vi "Open Session.vi"(6 "verify server (T)":bool=TRUE, 8 "error in":errorcluster, 9 "password":string, 10 "username":string, 11 "cookie file":path) -> (0 "error out":errorcluster, 3 "session":refnum<class "Session.lvclass">)   [LabVIEW 2024, in "lib_NI_Advanced HTTP Client.lvlib" / "Session.lvclass"]
doc: "Opens an HTTP client session. Use an HTTP client session to wire together multiple HTTP VIs while preserving authentication credentials, HTTP headers, and cookies."
uses:
  Session.lvclass
  Session.lvclass/Session.ctl
  lvwebclient_64.dll
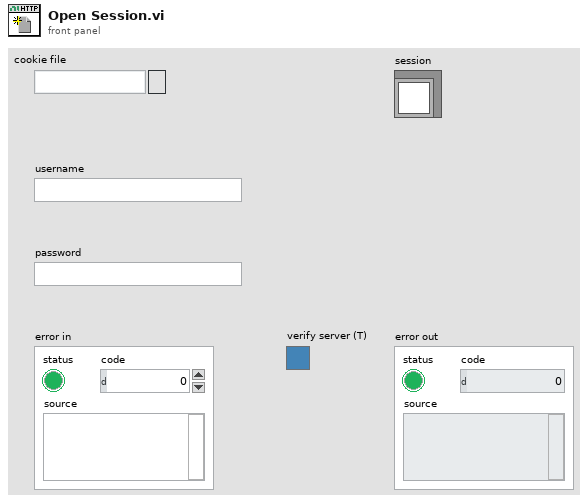
[diagram p1: front panel]
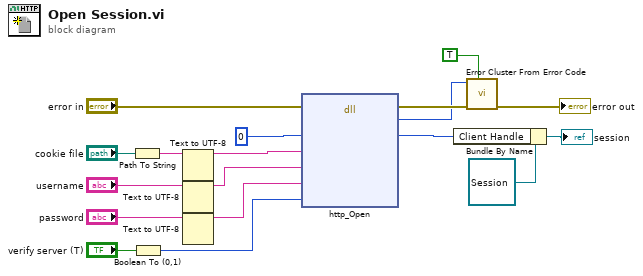
[diagram p0: block diagram]
diagram:
  n1 = Path To String(path="cookie file") -> (string=w6:string)
  n2 = Boolean To (0,1)(Boolean="verify server (T)") -> (0, 1=w12:i16)
  n3 = Text to UTF-8(11:w6) -> (3:w1:string)  [unwired: 2 in, 1 out]
  n4 = Text to UTF-8(11:"username") -> (3:w2:string)  [unwired: 2 in, 1 out]
  n5 = Text to UTF-8(11:"password") -> (3:w3:string)  [unwired: 2 in, 1 out]
  n6 = dll-call lib="C:/Program Files/National Instruments/LabVIEW 2024/vi.lib/NI/Advanced HTTP Client/lvwebclient_*.*" fn="http_Open"(error in="error in", "handle"=u32 0, "cookieFile"=w1, "username"=w2, "password"=w3, "verifyServer"=w12) -> (error out=w16:errorcluster, "return"=w14:i32, "handle"=w8:u32)  [unwired: 6 in, 1 out]
  n7 = Bundle By Name(cluster=refnum<class "Session.lvclass"> refnum ("HTTP Session"), "Client Handle"=w8) -> (→"session":refnum<class "Session.lvclass">)
  n8 = call "Error Cluster From Error Code.vi"("show call chain? (False)"=TRUE, "error in (no error)"=w16, "error code (0)"=w14) -> ("error out"=→"error out":errorcluster)  [unwired: 6 in]
